vi "BuildRelease_ParseStateQueue.vi"(0 "State Queue":string, 7 "Error In (no error)":errorcluster) -> (4 "Remaining States":string, 6 "Current State":string, 8 "Arguments":string)   [LabVIEW 2012]
doc: "Parses the State Machine state queue and returns the current state that will execute next with the associated arguments.\n\n<B>Inputs:</B>\n <B>State Queue:</B> The entire state queue is wired to this input. \n <B>Error In</B> The error cluster from the State Machine is wired to this input. If an error occures and appears on this input, the current state output returns the \"Error Handler\" state.\n\n<B>Outputs:</B>\n <B>Remaining States:</B> Returns all the next states that should execute after the current state completes. These should be passed through the current state in the state machine. These can also be modified or augmented within the current state if necessary.\n <B>Current State:</B> Returns the current state that should execute next in the state machine. If an error is wired to the Error input then the current state output becomes \"Error Handler\".\n <B>Arguments:</B> Returns any argument(s) that may be used in the current state string. These arguments come after the \">>\" characters. <B>Note:</B> The arguments variable must not contain any unprintable characters like linefeed or carriage return.\n\n<B>State Syntax:</B>\nStateCategory: State >> Argument\nLine Terminator: Line feed\n <B>Example:</B>\nUI: Help >> About\n\nWhere \"UI\" is the state category\nWhere \"Help\" is the state\nWhere \"About\" is the argument\n <B>Other Examples:</B>\nApp Data: Initialize\nUI: Initialize\nHelp >> About\n\n<B>Commenting:</B>\nTo add a comment use \"//\" or \"#\" and all text to the right will be ignored\n <B>Commenting Example:</B>\nUI: Initialize // This initializes the UI\n# This whole line is a comment\n// Another comment line"
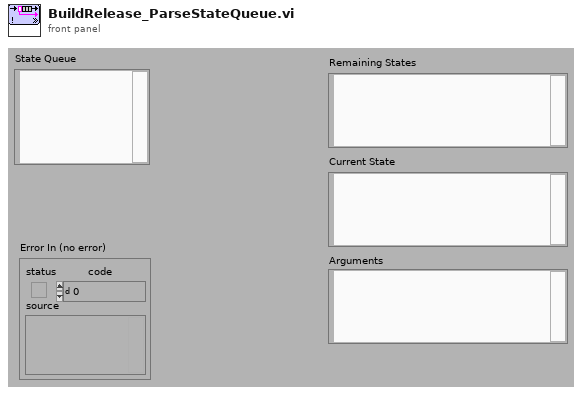
[diagram p1: front panel]
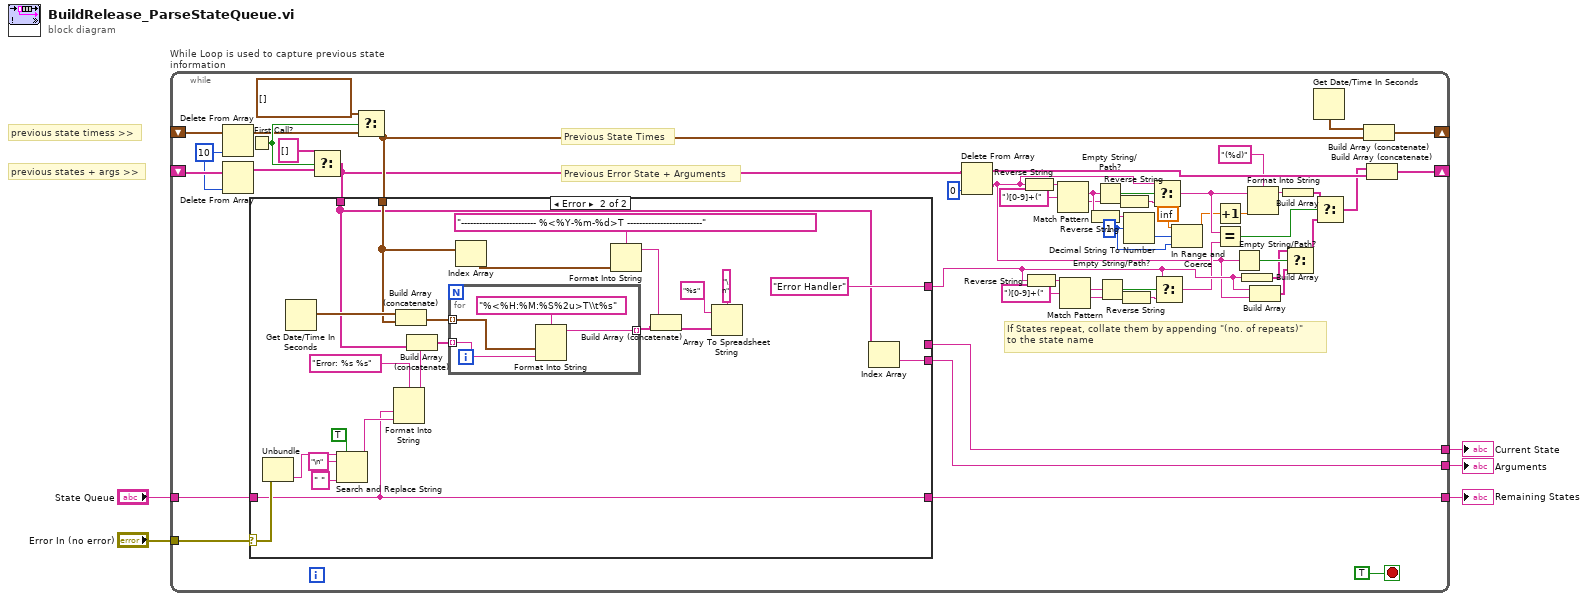
[diagram p0: block diagram]
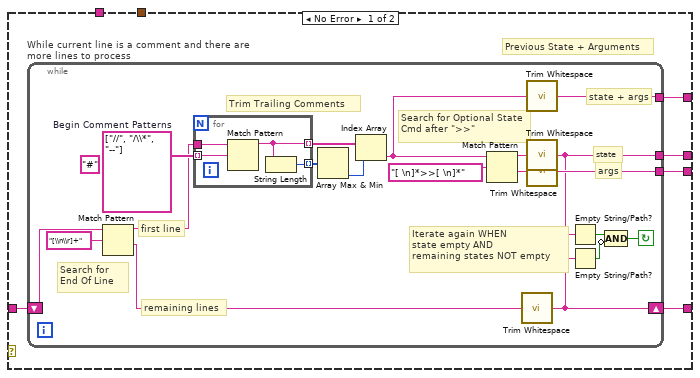
[diagram p2: hidden frame]
diagram:
  # "previous state timess >>"
  # "previous states + args >>"
  n1 = while "While Loop is used to capture previous state information" {
    tunnel: [w57] -> w5
    tunnel: "State Queue" -> [w56]
    tunnel: "Error In (no error)" -> [w55]
    tunnel: [w54] -> w2
    tunnel: [w53] -> w1
    shift-right: [w6] -> _
    shift-left: _ -> [w44]
    shift-right: [w50] -> _
    shift-left: _ -> [w46]
    stop <- TRUE stop-if-true
    w15 = 1 ("offset")
    w43 = 10 ("index")
    # "If States repeat, collate them by appending \"(no. of repeats)\"\nto the state name"
    # "Previous State Times"
    # "Previous Error State + Arguments"
    n2 = Delete From Array(array=w46, index=w43) -> (array with subset deleted=w45:timestamp[])  [unwired: 1 in, 1 out]
    n3 = Delete From Array(array=w44, index=w43) -> (array with subset deleted=w42:string[])  [unwired: 1 in, 1 out]
    n4 = First Call?() -> (First Call?: T/F=w48:bool)
    n5 = Select(t=string[] [], s=w48, f=w42) -> (s? t:f=w39:string[])
    n6 = Select(t=timestamp[] [], s=w48, f=w45) -> (s? t:f=w41:timestamp[])
    n7 = case shown="Error" w55 {
      selector: w55 -> [_ w95]
      tunnel: [w59 w88] -> w57
      tunnel: [w62 w108] -> w54
      tunnel: [w61 w86] -> w53
      tunnel: w56 -> [w60 w88]
      tunnel: [w58 w108] -> w40
      tunnel: w39 -> [_ w87]
      tunnel: w41 -> [_ w99]
      frame No Error {
        # "Previous State + Arguments"
        n8 = while "While current line is a comment and there are more lines to process" {
          tunnel: [w72] -> w62
          tunnel: [w73] -> w61
          shift-right: [w68] -> w59
          shift-left: w60 -> [w66]
          tunnel: [w63] -> w58
          stop <- w69 continue-if-true
          (unwired) "#"
          w80 = string[] ["//", "/\\*", "--"]  # Begin Comment Patterns
          # "state + args"
          # "remaining lines"
          # "first line"
          # "Search for End Of Line"
          # "Iterate again WHEN\nstate empty AND\nremaining states NOT empty"
          # "args"
          # "state"
          # "Search for Optional State Cmd after \">>\""
          # "Trim Trailing Comments"
          n9 = Match Pattern(string=w66, regular expression="[\\n\\r]+") -> (before substring=w65:string, after substring=w81:string)  [unwired: 3 out]
          n10 = for {
            tunnel: w65 -> [w85]
            tunnel: [w83] -> w77 mode=indexing
            tunnel: w80 -> [w84] mode=indexing
            tunnel: [w82] -> w79 mode=indexing
            n11 = Match Pattern(string=w85, regular expression=w84) -> (before substring=w83:string)  [unwired: 4 out]
            n12 = String Length(string=w83) -> (length=w82:i32)
          }
          n13 = Array Max & Min(array=w79) -> (min index (indices)=w78:i32)  [unwired: 3 out]
          n14 = Index Array(array=w77, index=w78) -> (element=w64:string)
          n15 = Match Pattern(string=w64, regular expression="[ \n]*>>[ \n]*") -> (before substring=w75:string, after substring=w74:string)  [unwired: 3 out]
          n16 = call <vilib>:"Trim Whitespace.vi"("string"=w81) -> ("trimmed string"=w68:string)  [unwired: 1 in]
          n17 = call <vilib>:"Trim Whitespace.vi"("string"=w64) -> ("trimmed string"=w63:string)  [unwired: 1 in]
          n18 = call <vilib>:"Trim Whitespace.vi"("string"=w75) -> ("trimmed string"=w72:string)  [unwired: 1 in]
          n19 = call <vilib>:"Trim Whitespace.vi"("string"=w74) -> ("trimmed string"=w73:string)  [unwired: 1 in]
          n20 = Empty String/Path?(string/path=w72) -> (empty?=w71:bool)
          n21 = Empty String/Path?(string/path=w68) -> (empty?=w70:bool)
          n22 = Compound Arithmetic op=AND(w71, invert w70) -> (w69:bool)
        }
      }
      frame Error {
        w108 = "Error Handler"
        n23 = Unbundle(w95) -> ("source"=w94:string)  [unwired: 2 out]
        n24 = Get Date/Time In Seconds() -> (seconds since 1Jan1904=w100:timestamp)
        n25 = Search and Replace String(replace all?=TRUE ("replace all? (F)"), input string=w94, search string="\n", replace string=" " ("replace string (\"\")")) -> (result string=w89:string)  [unwired: 1 in, 6 out]
        n26 = Format Into String(format string="Error: %s %s", w88, w89) -> (resulting string=w90:string)  [unwired: 2 in, 1 out]
        n27 = Build Array (concatenate)(w100, w99) -> (w98:timestamp[])
        n28 = Build Array (concatenate)(w90, w87) -> (w97:string[])
        n29 = for {
          tunnel: w97 -> [w110] mode=indexing
          tunnel: w98 -> [w111] mode=indexing
          tunnel: [w109] -> w102 mode=indexing
          n30 = Format Into String(format string="%<%H:%M:%S%2u>T\\t%s", w111, w110) -> (resulting string=w109:string)  [unwired: 2 in, 1 out]
        }
        n31 = Index Array(array=w99) -> (element=w104:timestamp)  [unwired: 1 in]
        n32 = Format Into String(format string="------------------------- %<%Y-%m-%d>T -------------------------", w104) -> (resulting string=w103:string)  [unwired: 2 in, 1 out]
        n33 = Build Array (concatenate)(w103, w102) -> (w101:string[])
        n34 = Array To Spreadsheet String(delimiter (Tab)="\n", array=w101, 3:"%s" ("format string")) -> ()  [unwired: 1 out]
        n35 = Index Array(array=w87) -> (element=w86:string)  [unwired: 1 in]
      }
    }
    n36 = Delete From Array(array=w39, index=0) -> (deleted portion=w10:string, array with subset deleted=w23:string[])  [unwired: 1 in]
    n37 = Reverse String(1:w10) -> (0:w38:string)
    n38 = Reverse String(1:w40) -> (0:w26:string)
    n39 = Match Pattern(string=w38, regular expression=")[0-9]+(") -> (match substring=w36:string, after substring=w34:string)  [unwired: 1 in, 2 out]
    n40 = Match Pattern(string=w26, regular expression=")[0-9]+(") -> (match substring=w28:string, after substring=w30:string)  [unwired: 1 in, 2 out]
    n41 = Reverse String(1:w36) -> (0:w32:string)
    n42 = Empty String/Path?(string/path=w36) -> (empty?=w35:bool)
    n43 = Empty String/Path?(string/path=w28) -> (empty?=w29:bool)
    n44 = Reverse String(1:w34) -> (0:w33:string)
    n45 = Reverse String(1:w30) -> (0:w31:string)
    n46 = Decimal String To Number(string=w32, offset=w15) -> (number=w16:i32)  [unwired: 1 in, 1 out]
    n47 = Select(t=w10, s=w35, f=w33) -> (s? t:f=w21:string)
    n48 = Select(t=w40, s=w29, f=w31) -> (s? t:f=w25:string)
    n49 = In Range and Coerce(upper limit=inf, x=w16, lower limit=w15) -> (coerced(x)=w13:dbl)  [unwired: 1 out]
    n50 = Increment(x=w13) -> (x+1=w20:dbl)
    n51 = Equal?(x=w21, y=w25) -> (x = y?=w12:bool)
    n52 = Empty String/Path?(string/path=w10) -> (empty?=w11:bool)
    n53 = Build Array(w40) -> (w7:string[])
    n54 = Format Into String(format string="(%d)" ("regular expression"), initial string=w21, w20) -> (resulting string=w18:string)  [unwired: 1 in, 1 out]
    n55 = Build Array(w40, w10) -> (w8:string[])
    n56 = Build Array(w18) -> (w17:string[])
    n57 = Select(t=w7, s=w11, f=w8) -> (s? t:f=w9:string[])
    n58 = Get Date/Time In Seconds() -> (seconds since 1Jan1904=w49:timestamp)
    n59 = Select(t=w17, s=w12, f=w9) -> (s? t:f=w22:string[])
    n60 = Build Array (concatenate)(w49, w41) -> (w50:timestamp[])
    n61 = Build Array (concatenate)(w22, w23) -> (w6:string[])
  }
  "Remaining States" <- w5
  "Arguments" <- w1
  "Current State" <- w2
